vi "delta_mn_zero.vi"(9 "fi":dbl, 10 "p":dbl, 11 "k":i32) -> (3 "y":dbl)   [LabVIEW 2020]
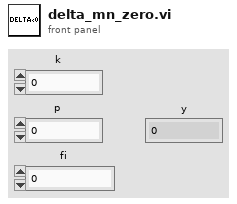
[diagram p1: front panel]
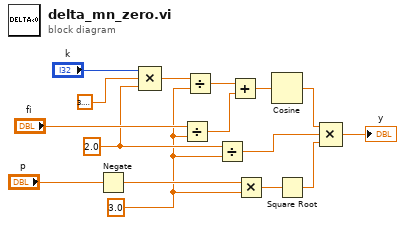
[diagram p0: block diagram]
diagram:
  w3 = 3.0 ("y")
  w5 = 2.0 ("x")
  n1 = Negate(x="p") -> (-x=w9:dbl)
  n2 = Compound Arithmetic op=MULTIPLY("k", 3.141592653589793, w5) -> (w2:dbl)
  n3 = Divide(x="fi", y=w3) -> (x/y=w4:dbl)
  n4 = Divide(x=w2, y=w3) -> (x/y=w1:dbl)
  n5 = Divide(x=w5, y=w3) -> (x/y=w6:dbl)
  n6 = Add(x=w1, y=w4) -> (x+y=w14:dbl)
  n7 = Multiply(x=w9, y=w3) -> (x*y=w10:dbl)
  n8 = Cosine(x=w14) -> (cos(x)=w15:dbl)
  n9 = Square Root(x=w10) -> (sqrt(x)=w7:dbl)
  n10 = Compound Arithmetic op=MULTIPLY(w15, w6, w7) -> (→"y":dbl)
